vi "Plug_in_data_global.vi"() -> ()   [LabVIEW 2010]
panel:
  in  "FFID Bkgnd Values":dbl[](array[numeric])
  in  "Templated Results header":string
  in  "Block Header":string
  in  "Server Channels to log":string[](array[string])
  in  "Vari Spaced":dbl[][](array[numeric]) format="%.2f"
  out "Second Plot data":cluster{"Xo":dbl, "Delta X":dbl, dbl[]}[](array[cluster]) {"?" format="%.2f"; "Delta X" format="%.2f"; "Xo" format="%.2f"}
  out "First Plot data":cluster{"Xo":dbl, "Delta X":dbl, dbl[]}[](array[cluster]) {"?" format="%.2f"; "Delta X" format="%.2f"; "Xo" format="%.2f"}
  in  "Voltages":dbl[][](array[numeric]) format="%.2f"
  in  "Analogue Binary":i16[][](array[numeric])
  in  "LDA Binary":u16[][](array[numeric])
  in  "Equi Spaced":dbl[][](array[numeric]) format="%.2f"
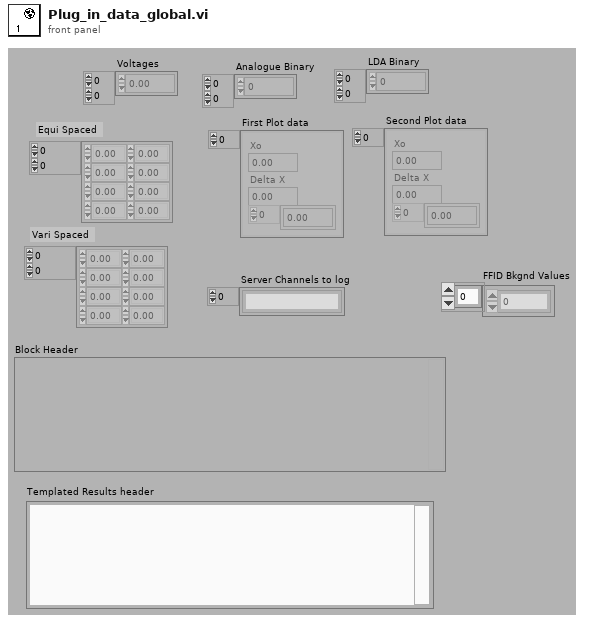
[diagram p1: front panel]
diagram:
